vi "getReportMsg.vi"(0 "partDescription":string, 1 "partNo":string, 2 "fixtureSerialNo":string, 3 "preparedBy":string, 4 "approvedBy":string, 5 "temprature":string, 6 "VNA Model:":enum16{"E5071C", "N5230A(C)", "N5224A", "9375A"}(ring)=enum."9375A", 8 "reportNo":string, 9 "application":string, 10 "sampleNo":string, 11 "rHumidity":string) -> (14 "value":string[](array[string]), 15 "item":string[](array[string])=["application", "partDescription", "partNo", "fixtureSerialNo", "reportNo", "sampleNo", "preparedBy", "approvedBy", "temprature", "rHumidity"])   [LabVIEW 2011]
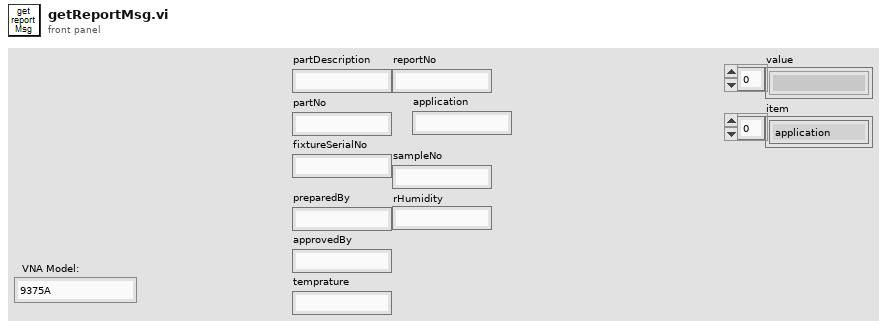
[diagram p1: front panel]
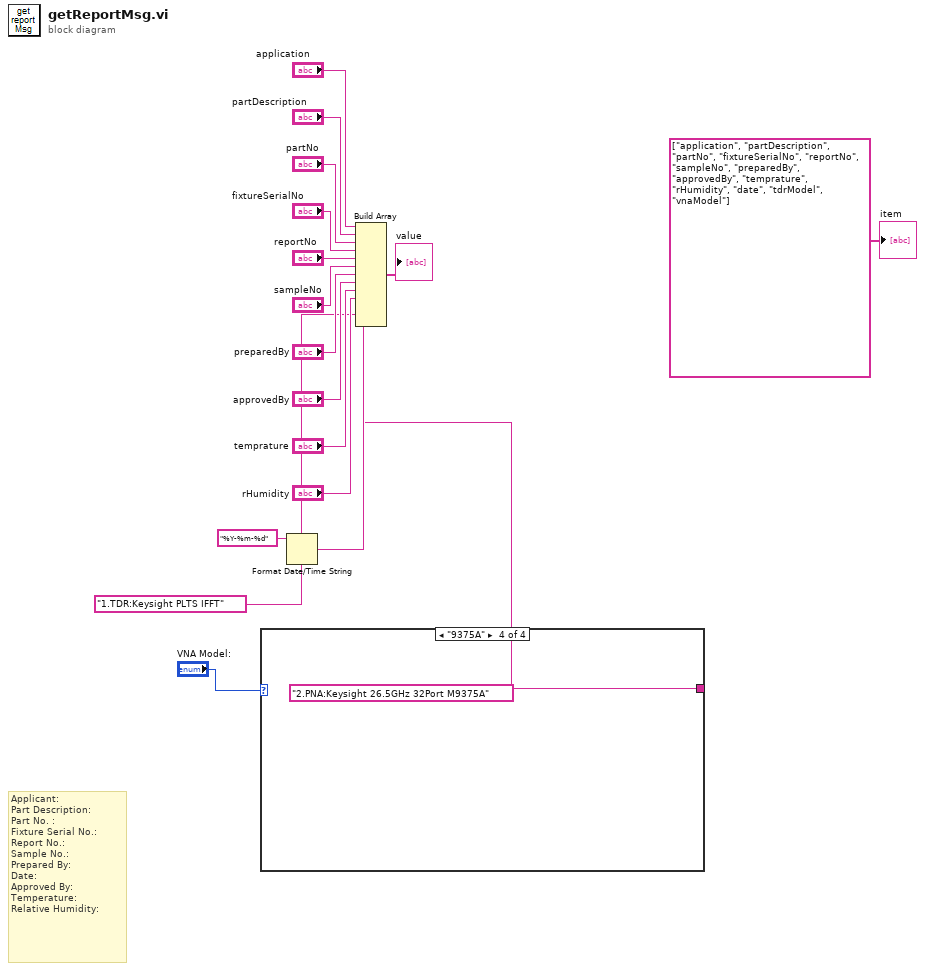
[diagram p0: block diagram]
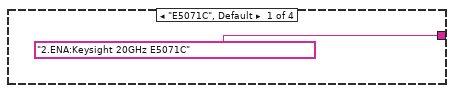
[diagram p2: hidden frame]
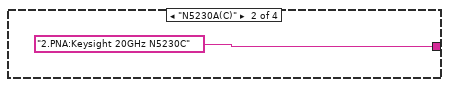
[diagram p3: hidden frame]
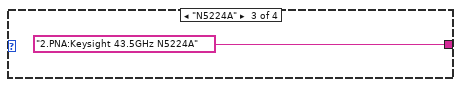
[diagram p4: hidden frame]
diagram:
  # "Applicant:\nPart Description:\nPart No. :\nFixture Serial No.:\nReport No.:\nSample No.:\nPrepared By:\nDate:\nApproved By:\nTemperature:\nRelative Humidity:"
  n1 = case shown="\"9375A\"" "VNA Model:" {
    tunnel: ["2.ENA:Keysight 20GHz E5071C" "2.PNA:Keysight 20GHz N5230C" "2.PNA:Keysight 43.5GHz N5224A" "2.PNA:Keysight 26.5GHz 32Port M9375A"] -> w1
    frame "E5071C", Default {
    }
    frame "N5230A(C)" {
    }
    frame "N5224A" {
    }
    frame "9375A" {
    }
  }
  n2 = Format Date/Time String(time format string (%c)="%Y-%m-%d" ("时间格式字符串(%c)")) -> (date/time string=w5:string)  [unwired: 2 in]
  n3 = Build Array("application", "partDescription", "partNo", "fixtureSerialNo", "reportNo", "sampleNo", "preparedBy", "approvedBy", "temprature", "rHumidity", w5, "1.TDR:Keysight PLTS IFFT" ("元素"), w1) -> (→"value":string[])
  "item" <- string[] ["application", "partDescription", "partNo", "fixtureSerialNo", "reportNo", "sampleNo", "preparedBy", "approvedBy", "temprature", "rHumidity", "date", "tdrModel", "vnaModel"]
